vi "PTScanner.constructor.vi"(0 "name":string, 2 "data in":string, 5 "error in(no error)":errorcluster) -> (14 "i ref out":refnum<vi>, 16 "data out":string, 19 "error out":errorcluster)   [LabVIEW 2014, in "PTScanner.lvlib"]
doc: "An event builder that collects data from DAQ devices and publishes them via DIM together with a description of the data.\n\nAn application sets a \"header\" of the data and the names of the DAQ devices by using the method \"Init\". When executing the method init, the EventBuilder will publish a DIM service \"EVENTBUILDERNAME_dataDesciption\" (see below).\n\nDuring data acquisition, three things happen.\n1) An applicatoin triggers the read out of the DAQ devices by using the command \"ReadDAQData\". This requires that an \"eventID\" is sent together with the \"ReadDAQData\" is incremented for each subsequent command.\n2) Then, the DataCollector will collect the data by queyring the DAQ devices using a \"ReadData\" event. \n3) Finally, the DataCollector will publish the collected event data as a DIM service \"EVENTBUILDERNAME_eventData\".\n\n\n\"EVENTBUILDERNAME_dataDescription\" has the format \"D:1;C:32768;C\" and contains a headerID (double timestamp), the names of the DAQ devices (char names[32768], names separated by \"|\") and a user defined data header (char *header).\n\n\"EVENTBUILDERNAME_eventData\" has the format \"D:1;D:1;L:1;C\" and contains the headerID (double timestamp), a timestamp (double timestamp), an eventID (long index) and the data (char *data). The data themselves are bundled using the \"data 2 bytea array\" from the CoreLib. Hence, they are packed according to the CS command format \"C:N;C:N;C:N[;C:N;C:N;C:N'[;...]]\", where the first string contains the name of the DAQDevice, the second string contains the \"data descriptor\" of the data and the last byte array contains the \"data\" according to the \"data descriptor\". Since there can be more than one DAQDevice, each set of even data may contain data of more than one DAQDevice.\n\nWARNING: It might be possible, that a client receives DIM service data more than once. As an example, this can happen, when a client re-connects to the DIM server publishing the data. In order to avoid duplicate data, the client MUST analyze the headerID (making sure, that the data belongs to the same \"run\") and the eventID (making sure, that no data is missed or duplicate).\n\nIMPORTANT: One must consider the size of the \"EVENTBUILDERNAME_eventData\" service. Typically, all DIM services are published in \"safe mode\", which means that subscribing to a DIM service that is published by the same OS-task will work. However, if one would like to publish large services, it might be necessary to disable the \"safe mode\". In that case a task must not subsribe to its own services. The \"safe mode\" can be enabled/disabled via the configuration database.\n\nauthor: Dietrich Beck, GSI\nmaintainer: Dietrich Beck, GSI\n\nLicense Agreement for this software:\n\nCopyright (C)\nGesellschaft für Schwerionenforschung, GSI\nPlanckstr. 1\n64291 Darmstadt\nGermany\n\nContact: D.Beck@gsi.de \n\nThis program is free software; you can redistribute it and/or modify it under the terms of the \nGNU General Public License as published by the Free Software Foundation; either version 2 of \nthe license, or (at your option) any later version.\n\nThis program is distributed in the hope that it will be useful, but WITHOUT ANY WARRANTY; \nwithout even the implied warranty of MERCHANTABILITY or FITNESS FOR A PARTICULAR PURPOSE. See the GNU General License for more details (http://www.gnu.org).\n\nGesellschaft für Schwerionenforschung, GSI\nPlanckstr. 1, 64291 Darmstadt, Germany\nFor all questions and ideas contact: M.Richter@gsi.de, H.Brand@gsi.de or D.Beck@gsi.de.\nLast update: 16-JUN-2004"
uses:
  PTScanner.lvlib
  CS_Core/BaseProcess/BaseProcess.lvlib
  CS_Core/CSSystem/CSSystemLib/CSSystemLib.lvlib
  CSlibraries-extern/DimLVEvent/LVDimInterface/LVDimInterface.lvlib
  CS_Core/BaseGUI/BaseGUI.lvlib
  CS_Core/CSObj/CSObj.lvlib
  CS_Core/BaseSM/BaseSM.lvlib
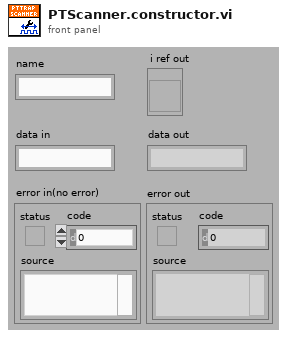
[diagram p1: front panel]
types:
  T1 = enum16{"SetAttribute", "GetAttribute", "CreateAttribute", "DestroyAttribute", "DestroyAllAtributes"}
  T2 = typedef "BaseProcess.lvlib/BaseProcess.i attribute.ctl" = cluster{"EventStatus":string, "EventError":i32, "PresetEvtWatchD":i32, "PresetPdcWatchD":i32, "EventTimeout":i32, "PeriodicInterval":i32, "Interface":string[], "Address":string[], "Special":string[], "PeriodicError":i32, "PeriodicStatus":string, "SuperProc":string, "Descriptors":T3[], "CaseRef":refnum<vi>, "PdcRef":refnum<vi>, "Thread Ref":refnum<vi>, "eventErrorID":i32, "eventStatusID":i32, "periodicErrorID":i32, "periodicStatusID":i32, "pdcCtrID":i32}
  T3 = typedef "BaseProcess.lvlib/BaseProcess.descriptor definition.ctl" = cluster{"selector":string, "descriptor":T4}
  T4 = typedef "BaseProcess.lvlib/BaseProcess.descriptor string definition.ctl" = string
  T5 = typedef "PTScanner.lvlib/PTScanner.i attribute.ctl" = cluster{"Object cmds":T6[], "Steps":cluster{"Finished":bool, "cmd setup":T7[]}[], "curStep":i32, "DIM IDs":cluster{"AllFinished":i32, "Finished":i32, "curStep":i32, "nofSteps":i32, "NomValues":i32[], "1D-Min":i32, "1D-Max":i32, "Dimensions":i32, "MaxDimensions":i32, "ScanedDeviceNames":i32[]}, "All Finished":bool, "DIMs in use":string[], "Running":bool, "Scan Delay":u32, "loop":bool, "Paused":bool, "Formed":bool}
  T6 = typedef "PTScanner.lvlib/PTScanner.obj parameters.ctl" = cluster{"object":string, "DIM address":string, "method":string, "data descriptor":string, "method parameters":cluster{"Name":string, "Descr":string, "Value":string, "Value?":bool}[], "Call Mode":enum16{"Simple DIM", "Synchronous"}, "actValue":dbl, "Centroid":dbl, "Minus Delta":dbl, "Plus Delta":dbl, "increment":dbl, "DIM Status":cluster{"no link":bool, "quality":i32, "Time Stamp":timestamp}, "range":dbl, "DIMChannelIndex":i32}
  T7 = typedef "PTScanner.lvlib/PTScanner.step obj parameters.ctl" = cluster{"obj index":i32, "nomValue":dbl, "fulfilled":bool}
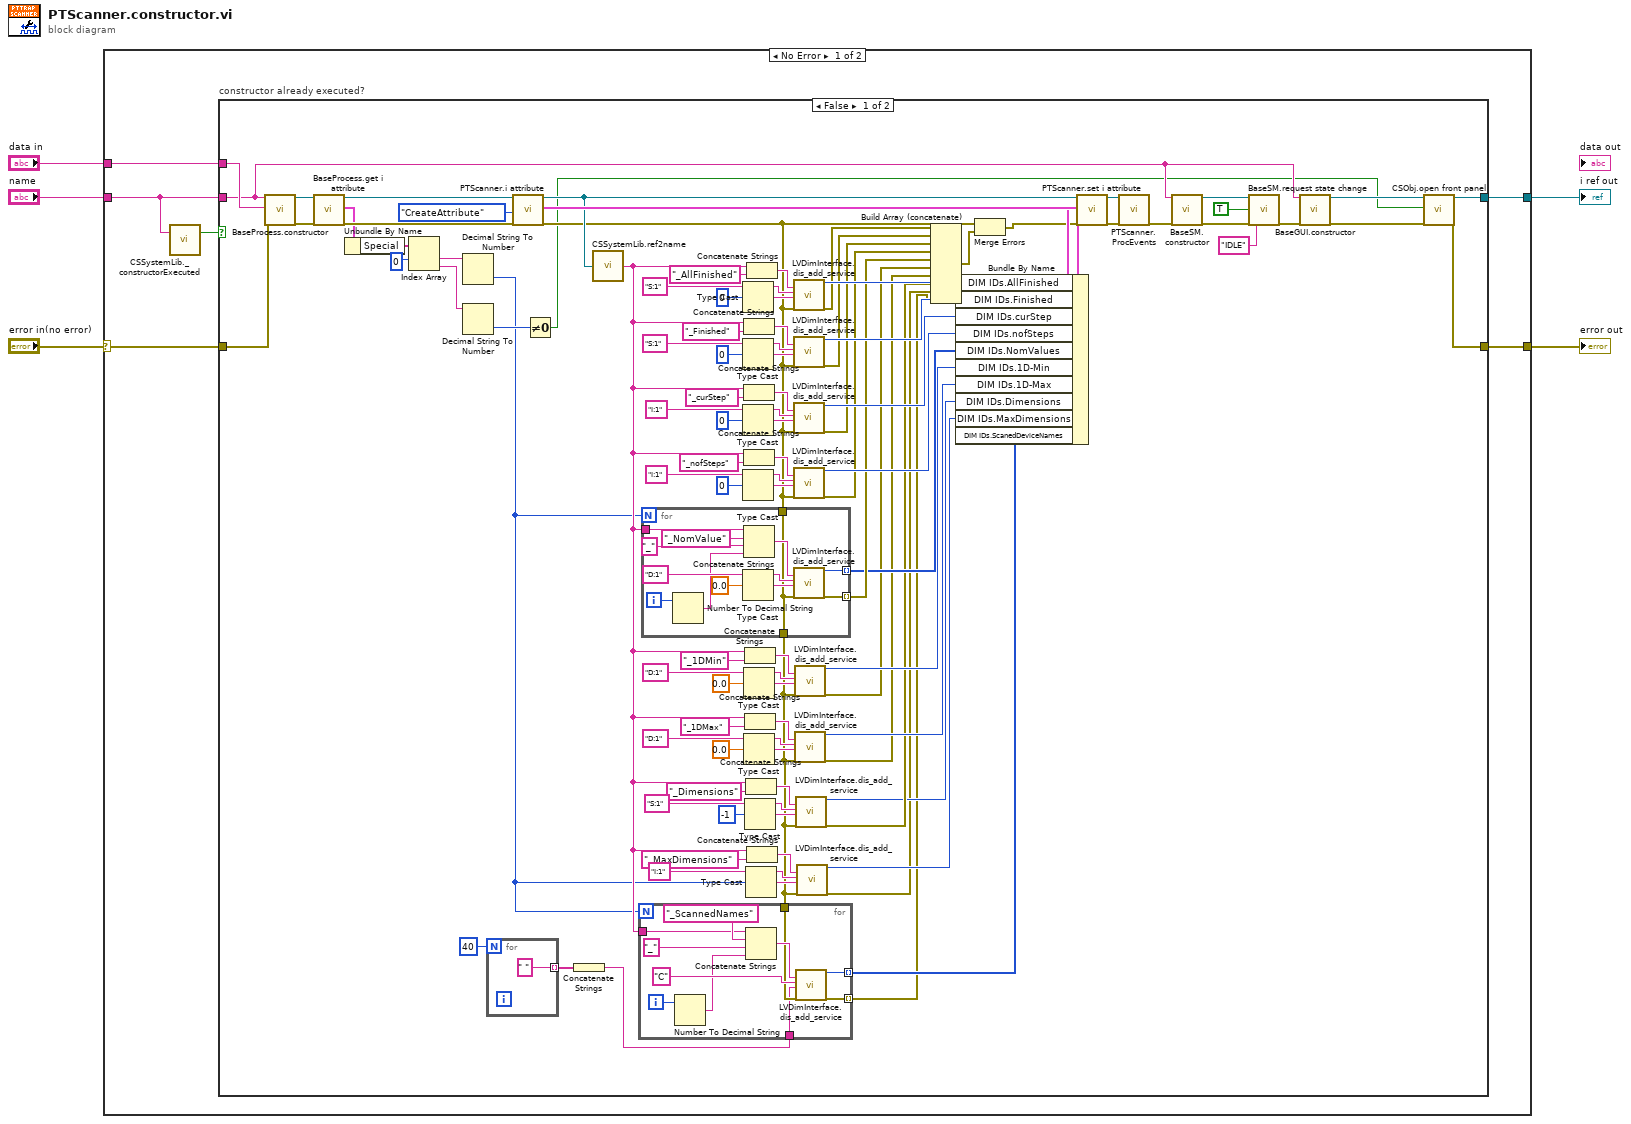
[diagram p0: block diagram]
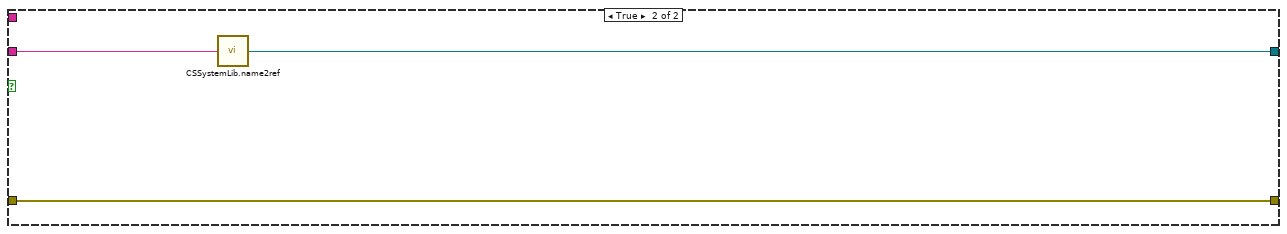
[diagram p2: hidden frame]
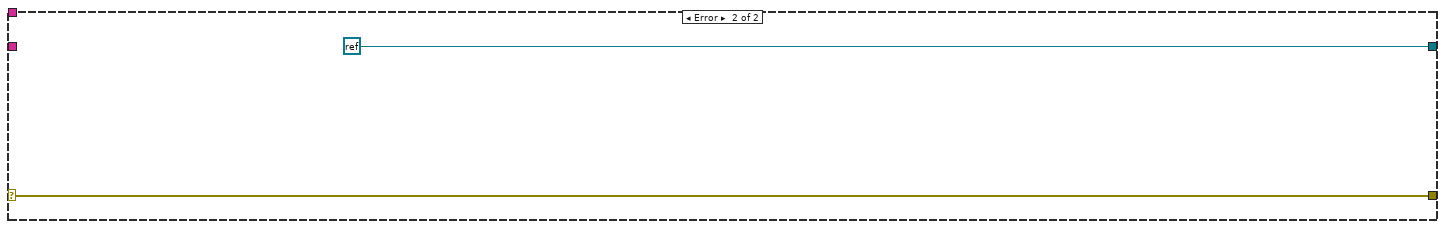
[diagram p3: hidden frame]
diagram:
  n1 = case shown="No Error" "error in(no error)" {
    selector: "error in(no error)" -> [w8 w137]
    tunnel: "name" -> [w6 _]
    tunnel: [w11 refnum<k0> refnum] -> w4
    tunnel: [w10 w137] -> w3
    tunnel: "data in" -> [w9 _]
    frame No Error {
      n2 = call "CSSystemLib._constructorExecuted.vi"("name"=w6) -> ("constructor executed?"=w7:bool)  [unwired: 18 in]
      n3 = case "constructor already executed?" shown="False" w7 {
        tunnel: w6 -> [w86 w136]
        tunnel: [w85 w135] -> w11
        tunnel: [w93 w134] -> w10
        tunnel: w9 -> [w108 _]
        tunnel: w8 -> [w107 w134]
        frame False {
          n4 = call "BaseProcess.constructor.vi"("name"=w86, "data in"=w108, "error in (no error)"=w107) -> ("i ref out"=w58:refnum<vi>, "error out"=w60:errorcluster)  [unwired: 14 in, 1 out]
          n5 = call "BaseProcess.get i attribute.vi"("i ref in"=w58, "error in (no error)"=w60) -> ("i ref out"=w57:refnum<vi>, "i attribute"=w56:T2, "error out"=w59:errorcluster)  [unwired: 15 in]
          n6 = Unbundle By Name(w56) -> ("Special"=w55:string[])
          n7 = Index Array(array=w55, index #1=0 ("index")) -> (element #1=w50:string, element #2=w22:string)  [unwired: 1 in]
          n8 = Decimal String To Number(string=w50) -> (number=w17:i32)  [unwired: 2 in, 1 out]
          n9 = Decimal String To Number(string=w22) -> (number=w21:i32)  [unwired: 2 in, 1 out]
          n10 = for {
            N: 40 -> [_]
            tunnel: [" "] -> w14 mode=indexing
          }
          n11 = call "PTScanner.i attribute.vi"("VI Refnum"=w57, "Action"=T1."CreateAttribute", "error in (no error)"=w59) -> ("VI Refnum out"=w84:refnum<vi>, "CLASS.i attribute out"=w97:T5, "error out"=w53:errorcluster)  [unwired: 14 in]
          n12 = Not Equal To 0?(x=w21) -> (x != 0?=w20:bool)
          n13 = Concatenate Strings(w14) -> (w13:string)
          n14 = call "CSSystemLib.ref2name.vi"("obj refnum"=w84) -> ("name"=w18:string)
          n15 = for {
            N: w17 -> [_]
            tunnel: w53 -> [w122]
            tunnel: [w128] -> w52 mode=indexing
            tunnel: w18 -> [w127]
            tunnel: [w123] -> w51 mode=indexing
            tunnel: [w122] -> w19
            i -> [w125]
            n16 = Number To Decimal String(number=w125) -> (decimal integer string=w124:string)  [unwired: 1 in]
            n17 = Type Cast(x=0.0) -> (*(type *) &x=w131:string)  [unwired: 1 in]
            n18 = Concatenate Strings(w127, "_NomValue", "_" ("string"), w124) -> (w130:string)
            n19 = call "LVDimInterface.dis_add_service.vi"("serviceName"=w130, "typeDescriptor"="D:1" ("initial string"), "data"=w131, "error in (no error)"=w122) -> ("my_serviceID"=w123:i32, "error out"=w128:errorcluster)  [unwired: 14 in]
          }
          n20 = for {
            N: w17 -> [_]
            tunnel: w19 -> [w112]
            tunnel: [w118] -> w15 mode=indexing
            tunnel: w18 -> [w117]
            tunnel: [w113] -> w16 mode=indexing
            tunnel: w13 -> [w111]
            i -> [w115]
            n21 = Number To Decimal String(number=w115) -> (decimal integer string=w114:string)  [unwired: 1 in]
            n22 = Concatenate Strings(w117, "_ScannedNames", "_" ("string"), w114) -> (w120:string)
            n23 = call "LVDimInterface.dis_add_service.vi"("serviceName"=w120, "typeDescriptor"="C" ("initial string"), "data"=w111, "error in (no error)"=w112) -> ("my_serviceID"=w113:i32, "error out"=w118:errorcluster)  [unwired: 14 in]
          }
          n24 = Type Cast(x=i16 0) -> (*(type *) &x=w104:string)  [unwired: 1 in]
          n25 = Type Cast(x=i16 0) -> (*(type *) &x=w102:string)  [unwired: 1 in]
          n26 = Type Cast(x=0) -> (*(type *) &x=w79:string)  [unwired: 1 in]
          n27 = Type Cast(x=0) -> (*(type *) &x=w71:string)  [unwired: 1 in]
          n28 = Concatenate Strings(w18, "_Finished") -> (w101:string)
          n29 = Concatenate Strings(w18, "_curStep") -> (w80:string)
          n30 = Concatenate Strings(w18, "_nofSteps") -> (w70:string)
          n31 = Type Cast(x=0.0) -> (*(type *) &x=w47:string)  [unwired: 1 in]
          n32 = Type Cast(x=0.0) -> (*(type *) &x=w41:string)  [unwired: 1 in]
          n33 = Concatenate Strings(w18, "_1DMin") -> (w46:string)
          n34 = Concatenate Strings(w18, "_1DMax") -> (w40:string)
          n35 = Type Cast(x=i16 -1) -> (*(type *) &x=w35:string)  [unwired: 1 in]
          n36 = Concatenate Strings(w18, "_Dimensions") -> (w34:string)
          n37 = Type Cast(x=w17) -> (*(type *) &x=w28:string)  [unwired: 1 in]
          n38 = Concatenate Strings(w18, "_AllFinished") -> (w103:string)
          n39 = Concatenate Strings(w18, "_MaxDimensions") -> (w27:string)
          n40 = call "LVDimInterface.dis_add_service.vi"("serviceName"=w103, "typeDescriptor"="S:1" ("initial string"), "data"=w104, "error in (no error)"=w53) -> ("my_serviceID"=w96:i32, "error out"=w64:errorcluster)  [unwired: 14 in]
          n41 = call "LVDimInterface.dis_add_service.vi"("serviceName"=w101, "typeDescriptor"="S:1" ("initial string"), "data"=w102, "error in (no error)"=w53) -> ("my_serviceID"=w95:i32, "error out"=w63:errorcluster)  [unwired: 14 in]
          n42 = call "LVDimInterface.dis_add_service.vi"("serviceName"=w80, "typeDescriptor"="I:1" ("initial string"), "data"=w79, "error in (no error)"=w53) -> ("my_serviceID"=w68:i32, "error out"=w62:errorcluster)  [unwired: 14 in]
          n43 = call "LVDimInterface.dis_add_service.vi"("serviceName"=w70, "typeDescriptor"="I:1" ("initial string"), "data"=w71, "error in (no error)"=w53) -> ("my_serviceID"=w67:i32, "error out"=w61:errorcluster)  [unwired: 14 in]
          n44 = call "LVDimInterface.dis_add_service.vi"("serviceName"=w46, "typeDescriptor"="D:1" ("initial string"), "data"=w47, "error in (no error)"=w19) -> ("my_serviceID"=w44:i32, "error out"=w37:errorcluster)  [unwired: 14 in]
          n45 = call "LVDimInterface.dis_add_service.vi"("serviceName"=w40, "typeDescriptor"="D:1" ("initial string"), "data"=w41, "error in (no error)"=w19) -> ("my_serviceID"=w38:i32, "error out"=w36:errorcluster)  [unwired: 14 in]
          n46 = call "LVDimInterface.dis_add_service.vi"("serviceName"=w34, "typeDescriptor"="S:1" ("initial string"), "data"=w35, "error in (no error)"=w19) -> ("my_serviceID"=w29:i32, "error out"=w30:errorcluster)  [unwired: 14 in]
          n47 = call "LVDimInterface.dis_add_service.vi"("serviceName"=w27, "typeDescriptor"="I:1" ("initial string"), "data"=w28, "error in (no error)"=w19) -> ("my_serviceID"=w24:i32, "error out"=w23:errorcluster)  [unwired: 14 in]
          n48 = Build Array (concatenate)(w64, w63, w62, w61, w52, w37, w36, w30, w23, w15) -> (w65:errorcluster[])
          n49 = Bundle By Name(cluster=w97, "DIM IDs.AllFinished"=w96, "DIM IDs.Finished"=w95, "DIM IDs.curStep"=w68, "DIM IDs.nofSteps"=w67, "DIM IDs.NomValues"=w51, "DIM IDs.1D-Min"=w44, "DIM IDs.1D-Max"=w38, "DIM IDs.Dimensions"=w29, "DIM IDs.MaxDimensions"=w24, "DIM IDs.ScanedDeviceNames"=w16) -> (w94:T5)
          n50 = Merge Errors(w53, w65) -> (w75:errorcluster)
          n51 = call "PTScanner.set i attribute.vi"("i ref in"=w84, "i attribute"=w94, "error in (no error)"=w75) -> ("i ref out"=w106:refnum<vi>, "error out"=w105:errorcluster)  [unwired: 15 in]
          n52 = call "PTScanner.ProcEvents.vi"("i ref in"=w106, "error in"=w105) -> ("error out"=w88:errorcluster)  [unwired: 16 in, 1 out]
          n53 = call "BaseSM.constructor.vi"("name"=w86, "error in (no error)"=w88) -> ("i ref out"=w89:refnum<vi>, "error out"=w90:errorcluster)  [unwired: 15 in, 1 out]
          n54 = call "BaseSM.request state change.vi"("i ref in"=w89, "change"=TRUE, "error in (no error)"=w90, "requested state"="IDLE") -> ("error out"=w87:errorcluster)  [unwired: 12 in, 3 out]
          n55 = call "BaseGUI.constructor.vi"("name"=w86, "error in (no error)"=w87) -> ("i ref out"=w83:refnum<vi>, "error out"=w82:errorcluster)  [unwired: 15 in, 1 out]
          n56 = call "CSObj.open front panel.vi"("i ref in"=w83, "frontPanelOpen"=w20, "error in (no error)"=w82) -> ("i ref out"=w85:refnum<vi>, "error out"=w93:errorcluster)  [unwired: 15 in]
        }
        frame True {
          n57 = call "CSSystemLib.name2ref.vi"("name"=w136) -> ("obj refnum"=w135:refnum<vi>)
        }
      }
    }
    frame Error {
    }
  }
  "i ref out" <- w4
  "error out" <- w3
